vi "Plotter_competition - file IO.vi"(8 "error in":errorcluster, 9 "Operation":T1(ring), 10 "File name":string, 11 "Data":dbl[](array[numeric])) -> (0 "error out":errorcluster)   [LabVIEW 2014]
doc: "Works as a functional global variable holding the file reference in memory using a shift register. Allows the program to create new folders and files on the U drive, write a binary file containing the data and then at the end of a run close the file."
panel:
  # "Inputs"
  # "Outputs"
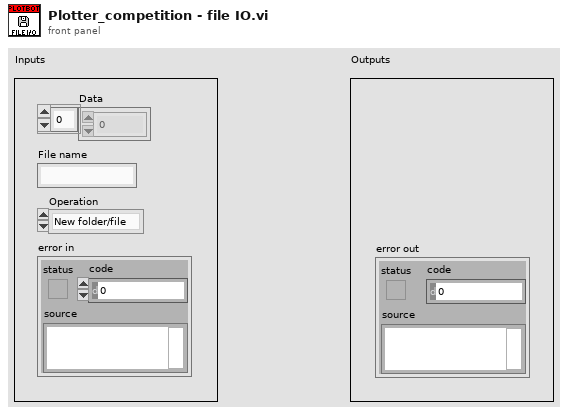
[diagram p1: front panel]
types:
  T1 = enum16{"New folder/file", "Create file", "Record", "Close"}
  T2 = enum16{"open", "replace", "create", "open or create", "replace or create", "replace or create with confirmation"}
  T3 = enum16{"big-endian, network order", "native, host order", "little-endian"}
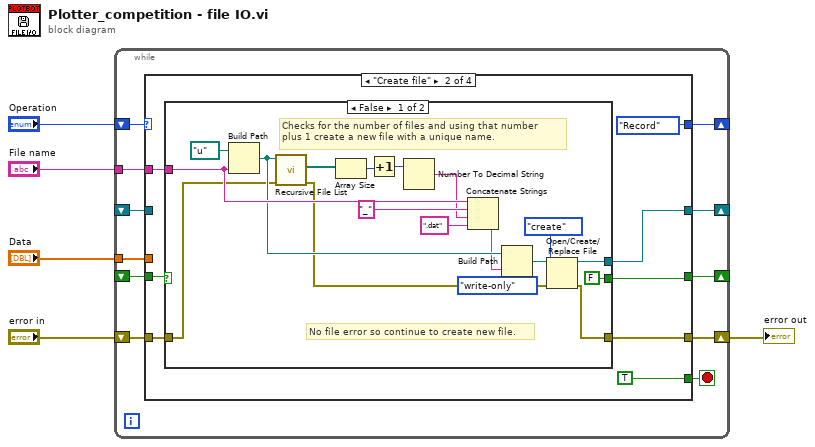
[diagram p0: block diagram]
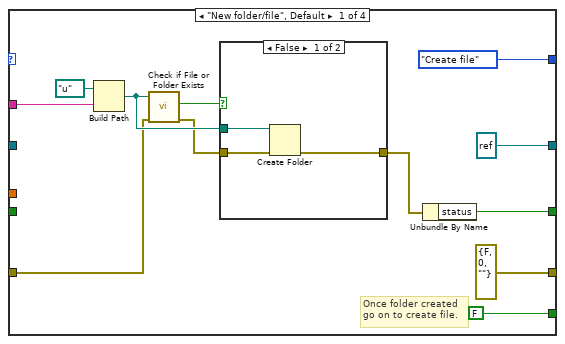
[diagram p2: hidden frame]
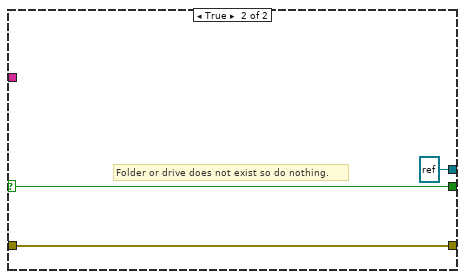
[diagram p4: hidden frame]
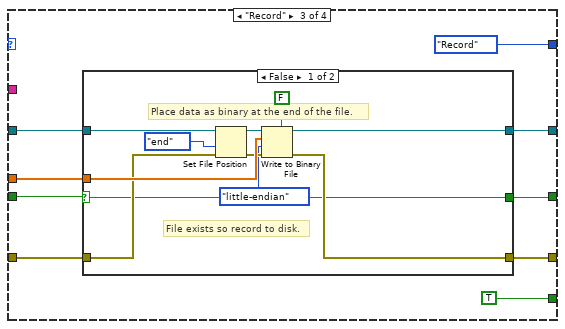
[diagram p5: hidden frame]
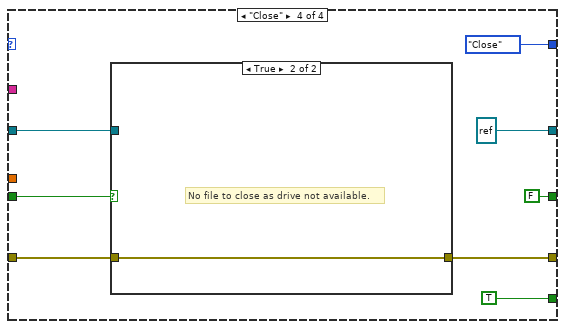
[diagram p7: hidden frame]
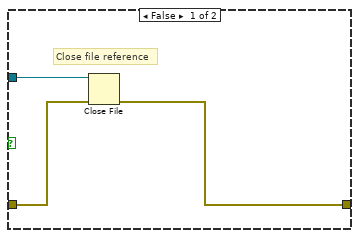
[diagram p8: hidden frame]
diagram:
  n1 = while {
    tunnel: "Data" -> [w16]
    shift-right: [w9] -> _
    shift-left: _ -> [w8]
    tunnel: "File name" -> [w14]
    shift-right: [w10] -> _
    shift-left: "Operation" -> [w15]
    shift-right: [w11] -> w1
    shift-left: "error in" -> [w13]
    shift-right: [w7] -> _
    shift-left: _ -> [w6]
    stop <- w12 stop-if-true
    n2 = case shown="\"Create file\"" w15 {
      tunnel: w16 -> [_ _ w68 _]
      tunnel: w14 -> [w28 w40 _ _]
      tunnel: w13 -> [w24 w38 w66 w91]
      tunnel: [FALSE TRUE TRUE TRUE] -> w12
      tunnel: [errorcluster {"status"=FALSE, "code"=0, "source"=""} ("error out") w37 w69 w90] -> w11
      tunnel: [T1."Create file" ("Operation") T1."Record" ("Operation") T1."Record" ("Operation") T1."Close" ("Operation")] -> w10
      tunnel: [refnum<file> refnum ("refnum out") w39 w70 refnum<file> refnum ("refnum out")] -> w9
      tunnel: w8 -> [_ _ w67 w92]
      tunnel: [w18 w33 w62 FALSE ("status")] -> w7
      tunnel: w6 -> [_ w34 w63 w86]
      frame "New folder/file", Default {
        # "Once folder created\ngo on to create file."
        n3 = Build Path(base path=path "u:/", name or relative path=w28) -> (appended path=w25:path)
        n4 = call <vilib>:"Check if File or Folder Exists.vi"("error in (no error)"=w24, "path"=w25) -> ("error out"=w23:errorcluster, "file or folder exists?"=w26:bool)  [unwired: 7 in, 1 out]
        n5 = case shown="False" w26 {
          tunnel: w25 -> [w31 _]
          tunnel: w23 -> [w30 w32]
          tunnel: [w29 w32] -> w19
          frame False {
            n6 = Create Folder(path (use dialog)=w31, error in=w30) -> (error out=w29:errorcluster)  [unwired: 1 in, 2 out]
          }
          frame True {
            # "Folder exists\nso don't create\na new one."
          }
        }
        n7 = Unbundle By Name(w19) -> ("status"=w18:bool)
      }
      frame "Create file" {
        n8 = case shown="False" w34 {
          selector: w34 -> [_ w59]
          tunnel: w40 -> [w56 _]
          tunnel: [w46 refnum<file> refnum ("refnum out")] -> w39
          tunnel: w38 -> [w45 w60]
          tunnel: [w43 w60] -> w37
          tunnel: [FALSE w59] -> w33
          frame False {
            # "No file error so continue to create new file."
            # "Checks for the number of files and using that number\nplus 1 create a new file with a unique name."
            n9 = Build Path(base path=path "u:/", name or relative path=w56) -> (appended path=w50:path)
            n10 = call <vilib>:"Recursive File List.vi"("error in (no error)"=w45, "Folder Path"=w50) -> ("error out"=w44:errorcluster, "All Files in Dir"=w57:path[])  [unwired: 5 in, 3 out]
            n11 = Array Size(array=w57) -> (size(s)=w54:i32)
            n12 = Increment(x=w54) -> (x+1=w53:i32)
            n13 = Number To Decimal String(number=w53) -> (decimal integer string=w52:string)  [unwired: 1 in]
            n14 = Concatenate Strings(w56, "_" ("string"), w52, ".dat" ("string")) -> (w49:string)
            n15 = Build Path(base path=w50, name or relative path=w49) -> (appended path=w48:path)
            n16 = Open/Create/Replace File(file path (use dialog)=w48, error in=w44, operation (0:open)=T2."create", access (0:read/write)=enum16{"read/write", "read-only", "write-only"}."write-only") -> (refnum out=w46:refnum<file>, error out=w43:errorcluster)  [unwired: 2 in, 1 out]
          }
          frame True {
            # "Folder or drive does not exist so do nothing."
          }
        }
      }
      frame "Record" {
        n17 = case shown="False" w63 {
          selector: w63 -> [w73 w84]
          tunnel: [w81 w83] -> w70
          tunnel: [w80 w82] -> w69
          tunnel: w68 -> [w79 _]
          tunnel: w67 -> [w77 w83]
          tunnel: w66 -> [w75 w82]
          tunnel: [w73 w84] -> w62
          frame False {
            # "File exists so record to disk."
            # "Place data as binary at the end of the file."
            n18 = Set File Position(refnum=w77, from (0:start)=enum16{"start", "end", "current"}."end", error in=w75) -> (refnum out=w76:refnum<file>, error out=w74:errorcluster)  [unwired: 1 in]
            n19 = Write to Binary File(file (use dialog)=w76, data=w79, error in=w74, 5:FALSE ("prepend array or string size? (T)"), 9:T3."little-endian" ("byte order (0:big-endian, network order)")) -> (refnum out=w81:refnum<file>, error out=w80:errorcluster)  [unwired: 1 in, 1 out]
          }
          frame True {
            # "No drive attached or folder created, do not write to file."
          }
        }
      }
      frame "Close" {
        n20 = case shown="True" w86 {
          tunnel: w92 -> [w95 _]
          tunnel: w91 -> [w94 w96]
          tunnel: [w93 w96] -> w90
          frame False {
            # "Close file reference"
            n21 = Close File(refnum=w95, error in=w94) -> (error out=w93:errorcluster)  [unwired: 1 out]
          }
          frame True {
            # "No file to close as drive not available."
          }
        }
      }
    }
  }
  "error out" <- w1
